vi "Write bt_Blackboard.vi"(8 "error in (no error)":errorcluster, 10 "Blackboard.lvclass":refnum<class "Blackboard.lvclass">, 11 "bt_WaitOn_Queue in":refnum<class "bt_WaitOn_Notifier.lvclass">) -> (0 "error out":errorcluster, 3 "bt_WaitOn_Queue out":refnum<class "bt_WaitOn_Notifier.lvclass">)   [LabVIEW 2021, in "BT.lvlib" / "bt_WaitOn_Notifier.lvclass"]
uses:
  bt_WaitOn_Notifier.lvclass
  bt_WaitOn_Notifier.lvclass/bt_WaitOn_Notifier.ctl
  Blackboard/Blackboard.lvclass
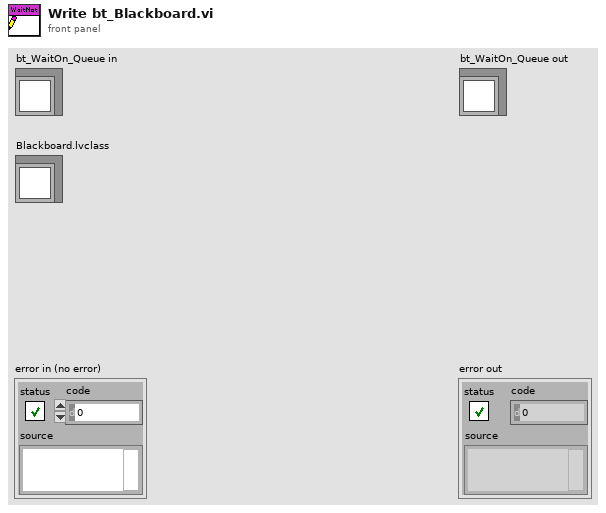
[diagram p1: front panel]
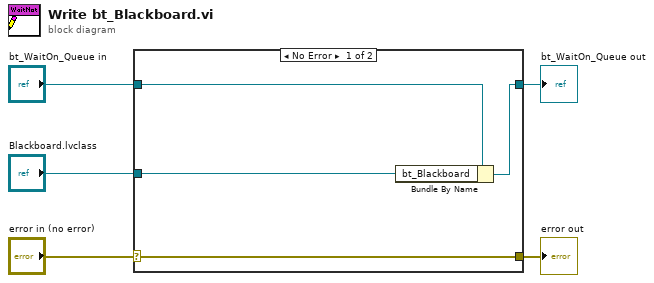
[diagram p0: block diagram]
diagram:
  n1 = case shown="No Error" "error in (no error)" {
    selector: "error in (no error)" -> [w9 w10]
    tunnel: [w9 w10] -> w4
    tunnel: [w7 w11] -> w2
    tunnel: "bt_WaitOn_Queue in" -> [w8 w11]
    tunnel: "Blackboard.lvclass" -> [w6 _]
    frame No Error {
      n2 = Bundle By Name(cluster=w8, "bt_Blackboard"=w6) -> (w7:refnum<class "bt_WaitOn_Notifier.lvclass">)
    }
    frame Error {
    }
  }
  "error out" <- w4
  "bt_WaitOn_Queue out" <- w2
